vi "Cleanup.vi"(8 "error in (no error)":errorcluster, 11 "Panel in":refnum<class "Panel.lvclass">) -> (0 "error out":errorcluster, 3 "Panel out":refnum<class "Panel.lvclass">)   [LabVIEW 2018, in "OOPanel.lvlib" / "Panel.lvclass"]
uses:
  Panel.lvclass
  Panel.lvclass/Panel.ctl
  Ref Data.ctl
  Panel Events.ctl
  Panel Visibility Changed.ctl
  State.ctl
  Desired Size.ctl
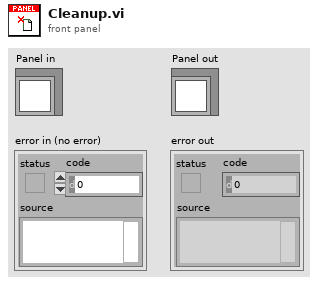
[diagram p1: front panel]
types:
  T1 = typedef "OOPanel.lvlib/Panel.lvclass/Ref Data.ctl" = cluster{"Panel VI":refnum<vi>, "Close":bool, "Panel Events":T2, "Running":bool, "Desired Size":T3, "Subpanel":refnum<vi>, "State":T4}
  T2 = typedef "OOPanel.lvlib/Panel.lvclass/Panel Events.ctl" = cluster{"Close":refnum<user-event>, "Visibility Changed":refnum<user-event>}
  T3 = typedef "OOPanel.lvlib/Panel.lvclass/Desired Size.ctl" = cluster{"Width":i16, "Height":i16}
  T4 = typedef "OOPanel.lvlib/Panel.lvclass/State.ctl" = enum16{"Idle", "Hidden", "Visible", "Subpanel"}
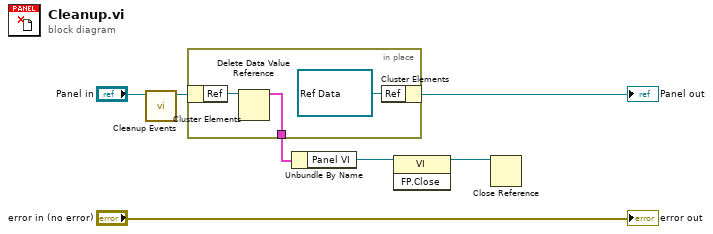
[diagram p0: block diagram]
diagram:
  n1 = call "Cleanup Events.vi"("Panel in"="Panel in") -> ("Panel out"=w6:refnum<class "Panel.lvclass">)  [unwired: 9 in, 1 out]
  n2 = in-place {
    in-place-border: [w8] -> w4
    n3 = in-place-cluster #1(w6) -> ("Ref"=w9:refnum<data-value>)
    n4 = Delete Data Value Reference(data value reference=w9) -> (data value=w8:T1)  [unwired: 1 in, 1 out]
    n5 = in-place-cluster #1("Ref"=refnum<data-value> refnum) -> (→"Panel out":refnum<class "Panel.lvclass">)
  }
  n6 = Unbundle By Name(w4) -> ("Panel VI"=w3:refnum<vi>)
  n7 = invoke class="VI" method="FP.Close"(reference=w3) -> (reference out=w2:refnum<vi>)  [unwired: 2 in, 2 out]
  n8 = Close Reference(reference=w2) -> ()  [unwired: 1 in, 1 out]
  "error out" <- "error in (no error)"
